vi "EXPRES Interface.vi"(8 "error in (no error)":errorcluster) -> (0 "error constant":errorcluster)   [LabVIEW 2016]
panel:
  in  "Stop Button":bool
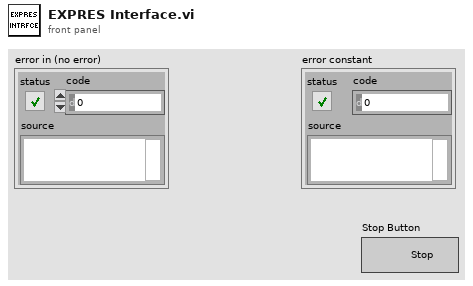
[diagram p1: front panel]
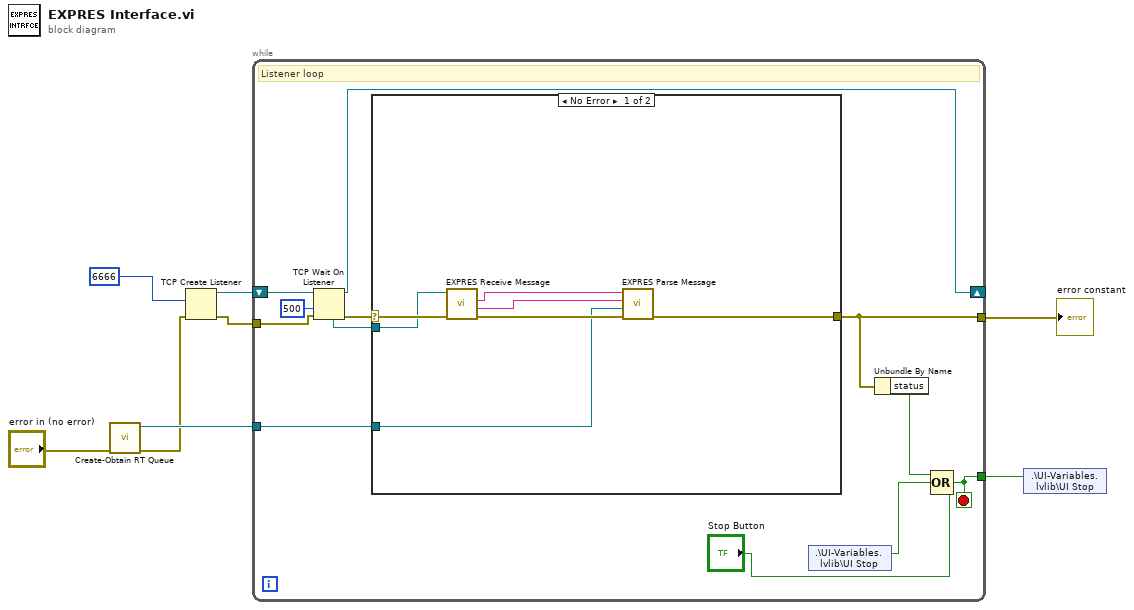
[diagram p0: block diagram]
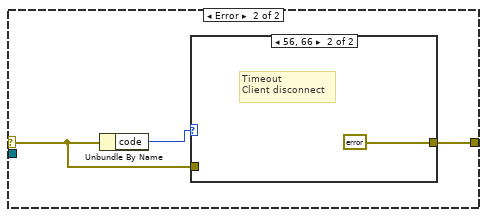
[diagram p2: hidden frame]
diagram:
  n1 = call "Create-Obtain RT Queue.vi"("error in (no error)"="error in (no error)") -> ("error out"=w1:errorcluster, "Queue out"=w3:refnum<queue>)  [unwired: 9 in]
  n2 = TCP Create Listener(8:w1, 10:u16 6666 ("port")) -> (0:w7:errorcluster, 3:w8:refnum<k5>)  [unwired: 3 in, 1 out]
  n3 = while {
    tunnel: [w20] -> w4
    tunnel: w7 -> [w15]
    shift-right: [w14] -> _
    shift-left: w8 -> [w18]
    tunnel: [w12] -> w5
    tunnel: w3 -> [w9]
    stop <- w20 stop-if-true
    # "Listener loop"
    n4 = TCP Wait On Listener(8:w15, 9:500 ("timeout ms (wait forever: -1)"), 11:w18) -> (0:w16:errorcluster, 3:w14:refnum<k5>, 4:w13:refnum<k5>)  [unwired: 1 in, 2 out]
    n5 = case shown="No Error" w16 {
      selector: w16 -> [w27 w29]
      tunnel: [w25 w28] -> w12
      tunnel: w13 -> [w26 _]
      tunnel: w9 -> [w21 _]
      frame No Error {
        n6 = call "EXPRES Receive Message.vi"("error in (no error)"=w27, "TCP Network Connection in"=w26) -> ("error out"=w24:errorcluster, "JSON string"=w22:string, "method"=w23:string)  [unwired: 6 in, 1 out]
        n7 = call "EXPRES Parse Message.vi"("error in (no error)"=w24, "queue"=w21, "JSON string"=w22, "method"=w23) -> ("error out"=w25:errorcluster)  [unwired: 7 in]
      }
      frame Error {
        n8 = Unbundle By Name(w29) -> ("code"=w30:i32)
        n9 = case shown="56, 66" w30 {
          tunnel: w29 -> [w31 _]
          tunnel: [w31 errorcluster {"status"=FALSE, "code"=0, "source"=""} ("error constant")] -> w28
          frame 0, Default {
          }
          frame 56, 66 {
            # "Timeout\nClient disconnect"
          }
        }
      }
    }
    n10 = shared-variable ".\\UI-Variables.lvlib\\UI Stop"() -> (w11:bool)  [unwired: 1 in, 1 out]
    n11 = Unbundle By Name(w12) -> ("status"=w19:bool)
    n12 = Compound Arithmetic op=OR(w19, w11, "Stop Button") -> (w20:bool)
  }
  "error constant" <- w5
  n13 = shared-variable ".\\UI-Variables.lvlib\\UI Stop"(w4) -> ()  [unwired: 1 in, 1 out]
